vi "SystemMessageDialogBox.vi"(6 "ErrorMessageToProcess":errorcluster, 8 "ErrorIn":errorcluster, 9 "CorrAct":string, 11 "Timeout":i32=-1) -> (0 "ErrorOut":errorcluster)   [LabVIEW 2018]
doc: "Call this modal dialog when an error occurs. This VI logs the error to a file to aid in diagnosis.\n\nThe CorrAct (Corrective Action) input can be used to suggest a solution to the user.\n\nCopyright © 2016 Epimedia, Inc. All Rights Reserved.\n\nThe Epimedia Application Library is Copyright © 2009-2016 Epimedia, Inc. \nAll Rights Reserved. Used under license."
uses:
  <vilib>/Utility/sysdir.llb/System Directory Type.ctl
panel:
  in  "Close":bool
  out "CorrAction":string caption="Corrective Action:"
  out "ErrorSource":string caption="Source:"
  out "ErrorCode":i32 caption="Code:"
  # "System Message"
  # "Copyright © 2016 Epimedia, Inc. All Rights Reserved.\n\nThe Epimedia Application Library is Copyright © 2009-2016 Epimedia, Inc. \nAll Rights Reserved. Used under license."
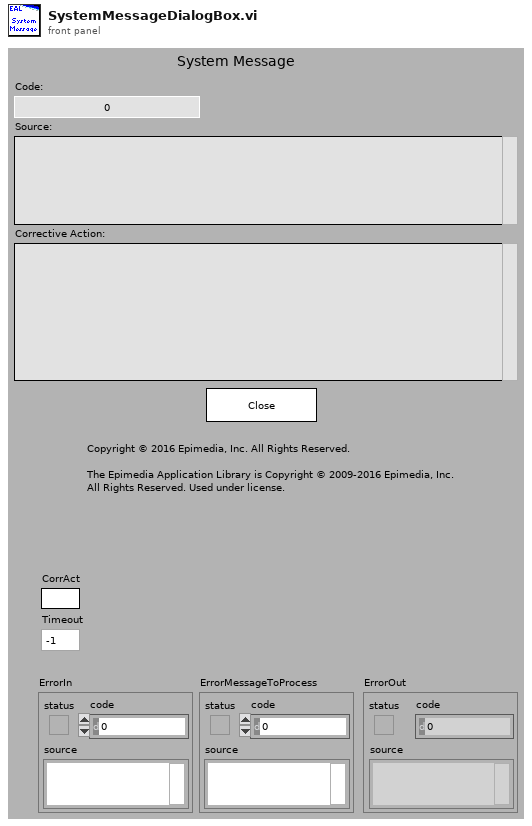
[diagram p1: front panel]
types:
  T1 = enum8{"Enabled", "Disabled", "Disabled and Grayed Out"}
  T2 = typedef "System Directory Type.ctl" = i32
  T3 = enum16{"open", "replace", "create", "open or create", "replace or create", "replace or create with confirmation"}
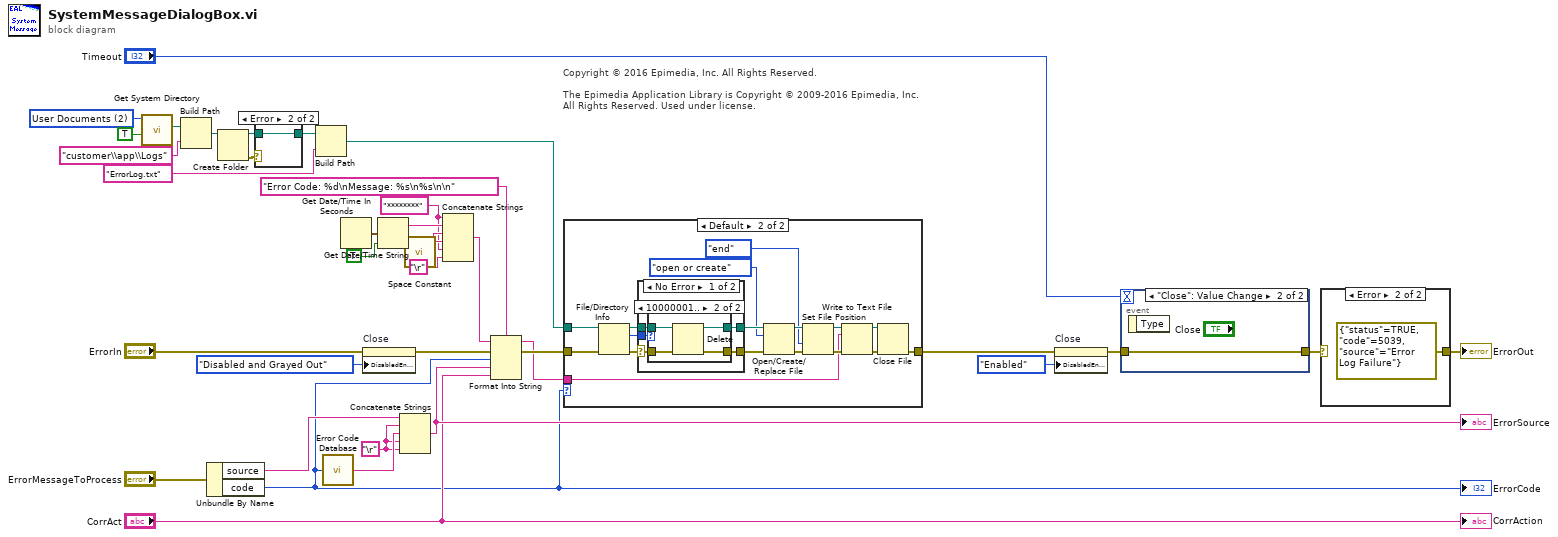
[diagram p0: block diagram]
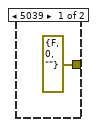
[diagram p2: hidden frame]
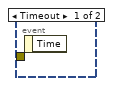
[diagram p7: hidden frame]
diagram:
  w25 = T2 2 items=["User Home"=0, "User Desktop"=1, "User Documents"=2, "User Application Data"=3, "User Preferences"=4, "User Temporary"=5, "Public Documents"=6, "Public Application Data"=7, "Public Preferences"=8, "Public Cache"=13, "System Core Libraries"=9, "System Installed Libraries"=10, "Application Files"=11, "Boot Volume Root"=12] ("system directory type")
  w28 = "********" ("string")
  w14 = "\r"
  # "Copyright © 2016 Epimedia, Inc. All Rights Reserved.\n\nThe Epimedia Application Library is Copyright © 2009-2016 Epimedia, Inc. \nAll Rights Reserved. Used under license."
  n1 = call <vilib>:"Get System Directory.vi"("create directory if not found? (F)"=TRUE, "system directory type"=w25) -> ("system directory"=w24:path)  [unwired: 9 in]
  n2 = Build Path(base path=w24, name or relative path="customer\\app\\Logs") -> (appended path=w17:path)
  n3 = Unbundle By Name("ErrorMessageToProcess") -> ("source"=w15:string, "code"=w1:i32)
  "ErrorCode" <- w1
  n4 = Create Folder(path (use dialog)=w17) -> (created path=w19:path, error out=w20:errorcluster)  [unwired: 2 in, 1 out]
  n5 = case shown="Error" w20 {
    tunnel: w19 -> [w38 w39]
    tunnel: [w38 w39] -> w18
    frame No Error {
    }
    frame Error {
    }
  }
  n6 = Build Path(base path=w18, name or relative path="ErrorLog.txt") -> (appended path=w16:path)
  n7 = call <vilib>:"Error Code Database.vi"("Error Code"=w1) -> ("Error Text"=w29:string)
  n8 = Get Date/Time In Seconds() -> (seconds since 1Jan1904=w36:timestamp)
  n9 = property on="Close" class="Bool"(error in="ErrorIn", "DisabledEnum"=T1."Disabled and Grayed Out" ("Disabled")) -> (error out=w4:errorcluster)  [unwired: 1 in, 1 out]
  n10 = Get Date/Time String(seconds (now)=w36, want seconds? (F)=TRUE) -> (date string=w35:string, time string=w34:string)  [unwired: 1 out]
  n11 = Concatenate Strings(w15, w14, w29, w14, w14) -> (w8:string)
  "ErrorSource" <- w8
  n12 = call <vilib>:"Space Constant.vi"() -> ("String"=w32:string)
  n13 = Concatenate Strings(w28, w35, w32, w34, w28, "\r") -> (w30:string)
  n14 = Format Into String(format string="Error Code: %d\nMessage: %s\n%s\n\n", initial string=w30, error in=w4, w1, w8, "CorrAct") -> (resulting string=w5:string, error out=w23:errorcluster)
  n15 = case shown="Default" w1 {
    tunnel: w23 -> [_ w44]
    tunnel: w16 -> [_ w43]
    tunnel: [errorcluster {"status"=FALSE, "code"=0, "source"=""} ("error out") w42] -> w10
    tunnel: w5 -> [_ w41]
    frame 5039 {
    }
    frame Default {
      n16 = File/Directory Info(path=w43, error in=w44) -> (path out=w54:path, size=w56:i64, error out=w57:errorcluster)  [unwired: 4 out]
      n17 = case shown="No Error" w57 {
        selector: w57 -> [w58 _]
        tunnel: [w62 _] -> w53
        tunnel: w54 -> [w61 w69]
        tunnel: [w60 w69] -> w55
        tunnel: w56 -> [w59 _]
        frame No Error {
          n18 = case shown="10000001.." w59 {
            tunnel: w58 -> [w63 w68]
            tunnel: [w63 w67] -> w62
            tunnel: w61 -> [w64 w66]
            tunnel: [w64 w65] -> w60
            frame ..10000000 {
            }
            frame 10000001.. {
              n19 = Delete(path (use dialog)=w66, error in=w68) -> (deleted path=w65:path, error out=w67:errorcluster)  [unwired: 3 in, 1 out]
            }
          }
        }
        frame Error {
        }
      }
      n20 = Open/Create/Replace File(file path (use dialog)=w55, error in=w53, operation (0:open)=T3."open or create") -> (refnum out=w50:refnum<file>, error out=w49:errorcluster)  [unwired: 4 out]
      n21 = Set File Position(refnum=w50, from (0:start)=enum16{"start", "end", "current"}."end", error in=w49) -> (refnum out=w51:refnum<file>, error out=w52:errorcluster)  [unwired: 1 out]
      n22 = Write to Text File(file (use dialog)=w51, text=w41, error in=w52) -> (refnum out=w47:refnum<file>, error out=w46:errorcluster)  [unwired: 2 out]
      n23 = Close File(refnum=w47, error in=w46) -> (error out=w42:errorcluster)  [unwired: 1 out]
    }
  }
  n24 = property on="Close" class="Bool"(error in=w10, "DisabledEnum"=T1."Enabled" ("Disabled")) -> (error out=w9:errorcluster)  [unwired: 1 in, 1 out]
  n25 = event shown="[1] \"Close\": Value Change" {
    selector: _ -> [_ _]
    dyn-events: _ -> [_ _]
    timeout: "Timeout" -> [_ _]
    tunnel: w9 -> [_ w70]
    tunnel: [_ w70] -> w3
    event Timeout {
      n26 = event-data() -> ()  [unwired: 2 out]
    }
    event "Close": Value Change {
      n27 = event-data() -> ()  [unwired: 2 out]
    }
  }
  n28 = case shown="Error" w3 {
    selector: w3 -> [w71 _]
    tunnel: [w71 errorcluster {"status"=TRUE, "code"=5039, "source"="Error Log Failure"} ("error IO")] -> w2
    frame No Error {
    }
    frame Error {
    }
  }
  "ErrorOut" <- w2
  "CorrAction" <- "CorrAct"
